vi "Interlock status global variable.vi"() -> ()   [LabVIEW 2020]
panel:
  out "Expt has Interlock?":bool
  in  "Experiment":string
  out "NOT SAFE":bool
  in  "Interlock Status":string
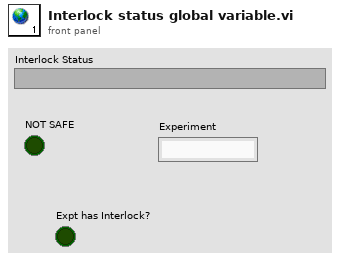
[diagram p1: front panel]
diagram:
